vi "niLvFpga_WaitOnIrq_cRIO-9034.vi"(0 "session in":u32, 5 "IRQ number mask":u32, 7 "timeout in ms":i32, 11 "error in":errorcluster) -> (4 "session out":u32, 6 "interrupt received?":bool, 8 "IRQs Asserted":u32, 10 "timed out?":bool, 15 "error out":errorcluster)   [LabVIEW 2017]
uses:
  <vilib>/rvi/interface/common/niFpgaWaitOnOcc.vi
  NiFpgaLv.dll
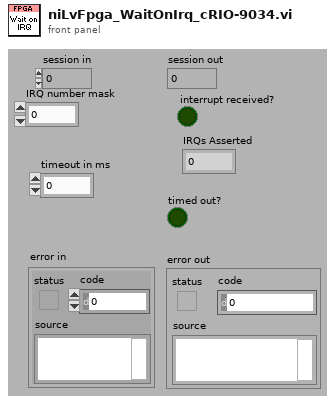
[diagram p1: front panel]
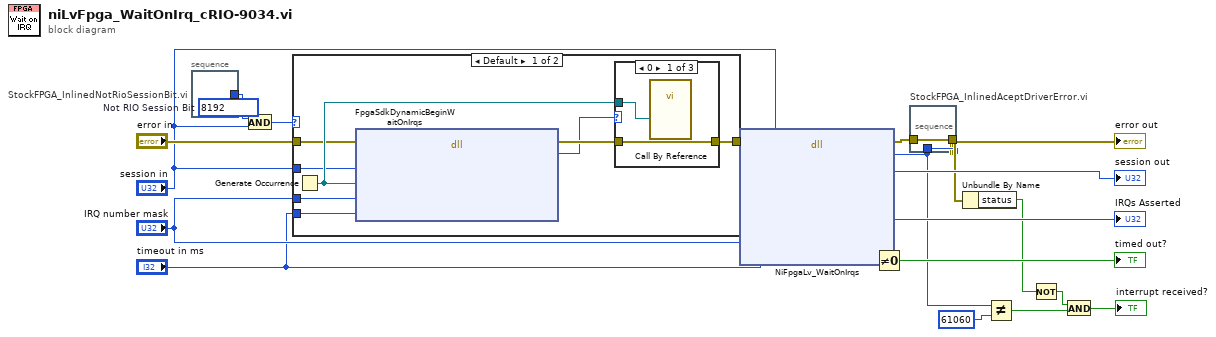
[diagram p0: block diagram]
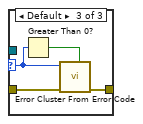
[diagram p4: hidden frame]
diagram:
  n1 = stacked-sequence "StockFPGA_InlinedNotRioSessionBit.vi" {
    tunnel: [w20] -> w7
    frame #0 {
      w20 = u32 8192  # Not RIO Session Bit
    }
  }
  n2 = And(x=w7, y="session in") -> (x .and. y?=w6:u32)
  n3 = case shown="Default" w6 {
    tunnel: "error in" -> [w25 w36]
    tunnel: [w24 w36] -> w4
    tunnel: "session in" -> [w23 _]
    tunnel: "IRQ number mask" -> [w22 _]
    tunnel: "timeout in ms" -> [w21 _]
    frame Default {
      n4 = Generate Occurrence() -> (w28:refnum<k4>)
      n5 = dll-call lib="LabVIEW" fn="FpgaSdkDynamicBeginWaitOnIrqs"(error in=w25, "session"=w23, "occurrence"=w28, "irqMask"=w22, "timeout"=w21) -> (error out=w27:errorcluster, "status"=w26:i32)  [unwired: 6 in, 1 out]
      n6 = case shown="0" w26 {
        selector: w26 -> [_ _ w32]
        tunnel: [w30 w31 w34] -> w24
        tunnel: w27 -> [w30 w31 w35]
        tunnel: w28 -> [w29 _ _]
        frame 0 {
          n7 = call-by-ref "?"("occurrence"=w29) -> ()  [unwired: 16 in, 3 out]
        }
        frame -61167 {
          # "emulation case intentionally ignoring error"
        }
        frame Default {
          n8 = Greater Than 0?(x=w32) -> (x > 0?=w33:bool)
          n9 = call <vilib>:"Error Cluster From Error Code.vi"("is warning? (False)"=w33, "error in (no error)"=w35, "error code (0)"=w32) -> ("error out"=w34:errorcluster)  [unwired: 6 in]
        }
      }
    }
    frame 0 {
    }
  }
  n10 = dll-call lib="NiFpgaLv.*" fn="NiFpgaLv_WaitOnIrqs" label="niLvFpgaWaitOnIRQ"(error in=w4, "sessionID"="session in", "irqs"="IRQ number mask", "timeout"="timeout in ms") -> (error out=w19:errorcluster, "status"=w14:i32, "sessionID"=→"session out":u32, "irqsAsserted"=→"IRQs Asserted":u32, "timedOut"=w16:u8)  [unwired: 5 in, 4 out]
  n11 = Not Equal To 0?(x=w16) -> (x != 0?=→"timed out?":bool)
  n12 = stacked-sequence "StockFPGA_InlinedAceptDriverError.vi" {
    tunnel: w19 -> [w37]
    tunnel: w14 -> [w39]
    tunnel: [w38] -> w12
    frame #0 {
      n13 = case shown="Default" w39 {
        selector: w39 -> [_ w41]
        tunnel: [w40 w43] -> w38
        tunnel: w37 -> [w40 w44]
        frame 0 {
        }
        frame Default {
          n14 = Greater Than 0?(x=w41) -> (x > 0?=w42:bool)
          n15 = call <vilib>:"Error Cluster From Error Code.vi"("is warning? (False)"=w42, "error in (no error)"=w44, "error code (0)"=w41) -> ("error out"=w43:errorcluster)  [unwired: 6 in]
        }
      }
    }
  }
  "error out" <- w12
  n16 = Unbundle By Name(w12) -> ("status"=w8:bool)
  n17 = Not Equal?(x=w14, y=61060) -> (x != y?=w11:bool)
  n18 = Not(x=w8) -> (.not. x?=w9:bool)
  n19 = And(x=w9, y=w11) -> (x .and. y?=→"interrupt received?":bool)
